vi "Facade Graph.vi"(0 "Data In":T4, 2 "Display State In":T2, 3 "Container State":T3) -> (6 "Data Out":T4, 7 "Display State Out":T2, 8 "Action":T1)   [LabVIEW 2009, in "Xgraph simple.xctl"]
doc: "Demonstration of an XControl.\n\nAAL 9/09"
uses:
  Xgraph simple.xctl
  Data Graph.ctl
  <vilib>/_xctls/Container State.ctl
  State Graph.ctl
  <vilib>/_xctls/Action.ctl
  <vilib>/_xctls/XControlSupport.lvlib
panel:
  in  "Plot Colors":u32[](array[colorbox])
  out "Xgraph simple":dbl[][](graph)
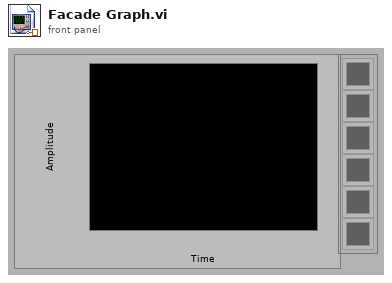
[diagram p1: front panel]
types:
  T1 = typedef "XControlSupport.lvlib/Action.ctl" = cluster{"Data Changed?":bool, "State Changed?":bool, "Action Name":string}
  T2 = typedef "Xgraph simple.xctl/State Graph.ctl" = cluster{"Show Points?":bool}
  T3 = typedef "XControlSupport.lvlib/Container State.ctl" = cluster{"Indicator?":bool, "Run Mode?":bool, " Refnum":refnum<vi>}
  T4 = typedef "Xgraph simple.xctl/Data Graph.ctl" = dbl[][]
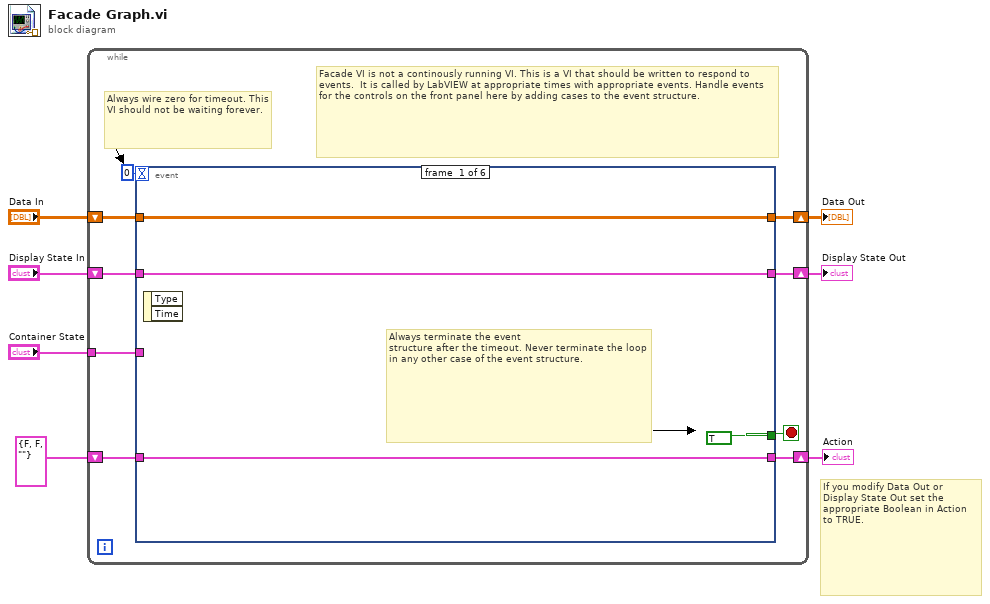
[diagram p0: block diagram]
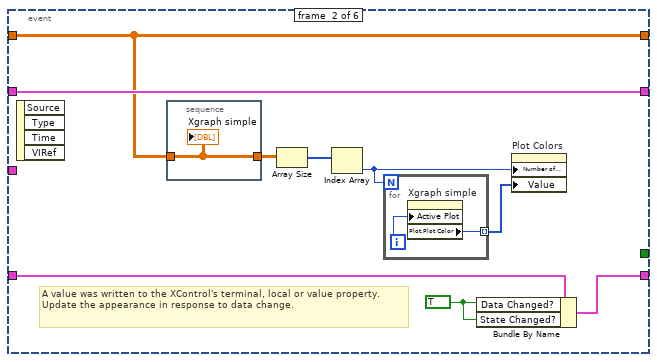
[diagram p2: hidden frame]
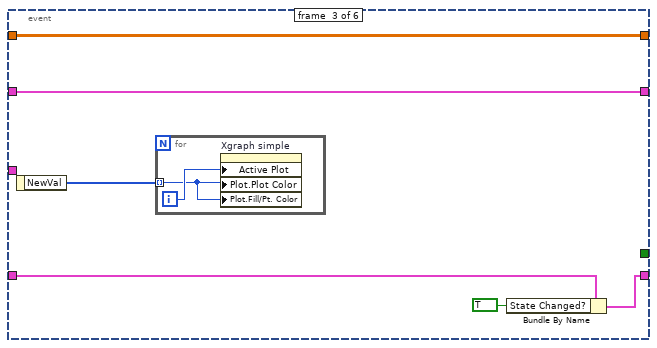
[diagram p3: hidden frame]
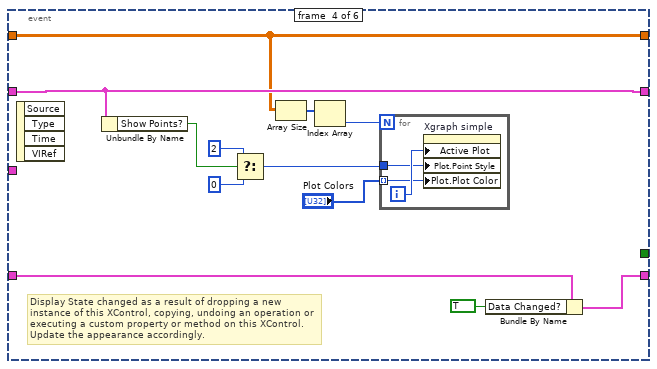
[diagram p4: hidden frame]
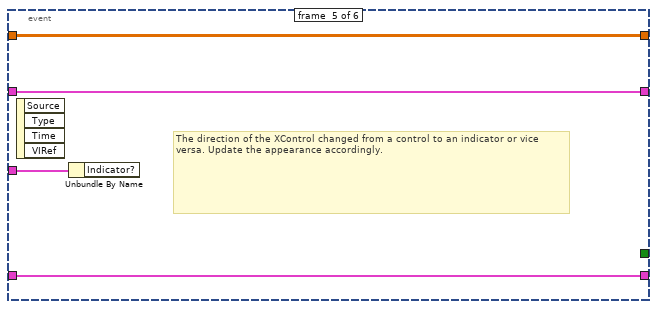
[diagram p5: hidden frame]
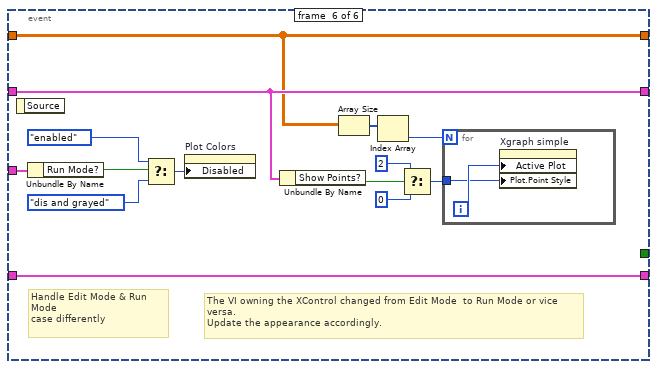
[diagram p6: hidden frame]
diagram:
  # "If you modify Data Out or\nDisplay State Out set the\nappropriate Boolean in Action\nto TRUE."
  n1 = while {
    shift-right: [w15] -> w4
    shift-left: "Display State In" -> [w16]
    tunnel: "Container State" -> [w12]
    shift-right: [w10] -> w7
    shift-left: "Data In" -> [w11]
    shift-right: [w8] -> w2
    shift-left: T1 {"Data Changed?"=FALSE, "State Changed?"=FALSE, "Action Name"=""} ("Action") -> [w9]
    stop <- w14 stop-if-true
    # "Facade VI is not a continously running VI. This is a VI that should be written to respond to events.  It is called by LabVIEW at appropriate times with appropriate events. Handle events for the controls on the front panel here by adding cases to the event structure."
    # "Always wire zero for timeout. This\nVI should not be waiting forever."
    n2 = event shown="[5] Exec State Change" {
      selector: _ -> [_ _ _ _ _ _]
      dyn-events: _ -> [_ _ _ _ _ _]
      timeout: 0 -> [_ _ _ _ _ _]
      tunnel: w16 -> [w18 w29 w33 w49 w58 w61]
      tunnel: [w18 w29 w33 w49 w58 w61] -> w15
      tunnel: [TRUE _ _ _ _ _] -> w14
      tunnel: w12 -> [_ _ _ _ w59 w73]
      tunnel: w11 -> [w17 w24 w35 w48 w57 w60]
      tunnel: [w17 w24 w35 w48 w57 w60] -> w10
      tunnel: [w19 w27 w37 w51 w56 w72] -> w8
      tunnel: w9 -> [w19 w28 w38 w52 w56 w72]
      event #0 {
        # "Always terminate the event\nstructure after the timeout. Never terminate the loop in any other case of the event structure."
        n3 = event-data() -> ()  [unwired: 1 in, 2 out]
      }
      event #1 {
        w26 = TRUE ("Data Changed?")
        # "A value was written to the XControl's terminal, local or value property.\nUpdate the appearance in response to data change."
        n4 = event-data() -> ()  [unwired: 1 in, 4 out]
        n5 = stacked-sequence {
          tunnel: w24 -> [w32]
          tunnel: [w32] -> w23
          frame #0 {
            "Xgraph simple" <- w32
          }
        }
        n6 = Array Size(array=w23) -> (size(s)=w25:i32[])
        n7 = Index Array(array=w25) -> (element=w22:i32)  [unwired: 1 in]
        n8 = for {
          N: w22 -> [_]
          tunnel: [w30] -> w21 mode=indexing
          i -> [w31]
          n9 = property on="Xgraph simple" class="WFGraph (strict)"("Active Plot"=w31) -> ("Plot.Plot Color"=w30:u32)  [unwired: 2 in, 2 out]
        }
        n10 = Bundle By Name(cluster=w28, "Data Changed?"=w26, "State Changed?"=w26) -> (w27:T1)
        n11 = property on="Plot Colors" class="Arr (strict)"("Number of Rows"=w22, "Value"=w21) -> ()  [unwired: 2 in, 2 out]
      }
      event #2 {
        n12 = event-data() -> ("NewVal"=w34:u32[])  [unwired: 1 in]
        n13 = for {
          tunnel: w34 -> [w39] mode=indexing
          i -> [w40]
          n14 = property on="Xgraph simple" class="WFGraph (strict)"("Active Plot"=w40, "Plot.Plot Color"=w39, "Plot.Fill/Pt. Color"=w39) -> ()  [unwired: 2 in, 2 out]
        }
        n15 = Bundle By Name(cluster=w38, "State Changed?"=TRUE) -> (w37:T1)
      }
      event #3 {
        # "Display State changed as a result of dropping a new instance of this XControl, copying, undoing an operation or executing a custom property or method on this XControl. Update the appearance accordingly."
        n16 = event-data() -> ()  [unwired: 1 in, 4 out]
        n17 = Unbundle By Name(w49) -> ("Show Points?"=w45:bool)
        n18 = Select(t=2, s=w45, f=0) -> (s? t:f=w42:i32)
        n19 = Array Size(array=w48) -> (size(s)=w47:i32[])
        n20 = Index Array(array=w47) -> (element=w46:i32)  [unwired: 1 in]
        n21 = for {
          N: w46 -> [_]
          tunnel: w42 -> [w54]
          tunnel: "Plot Colors" -> [w53] mode=indexing
          i -> [w55]
          n22 = property on="Xgraph simple" class="WFGraph (strict)"("Active Plot"=w55, "Plot.Point Style"=w54, "Plot.Plot Color"=w53) -> ()  [unwired: 2 in, 2 out]
        }
        n23 = Bundle By Name(cluster=w52, "Data Changed?"=TRUE) -> (w51:T1)
      }
      event #4 {
        # "The direction of the XControl changed from a control to an indicator or vice versa. Update the appearance accordingly."
        n24 = event-data() -> ()  [unwired: 1 in, 4 out]
        n25 = Unbundle By Name(w59) -> ()  [unwired: 1 out]
      }
      event #5 {
        # "The VI owning the XControl changed from Edit Mode  to Run Mode or vice versa.\nUpdate the appearance accordingly."
        # "Handle Edit Mode & Run Mode\ncase differently"
        n26 = event-data() -> ()  [unwired: 1 in, 1 out]
        n27 = Unbundle By Name(w73) -> ("Run Mode?"=w71:bool)
        n28 = Select(t=enum16{"enabled", "disabled", "dis and grayed"}."enabled", s=w71, f=enum16{"enabled", "disabled", "dis and grayed"}."dis and grayed") -> (s? t:f=w69:enum16{"enabled", "disabled", "dis and grayed"})
        n29 = property on="Plot Colors" class="Arr (strict)"("Disabled"=w69) -> ()  [unwired: 2 in, 2 out]
        n30 = Unbundle By Name(w61) -> ("Show Points?"=w65:bool)
        n31 = Array Size(array=w60) -> (size(s)=w67:i32[])
        n32 = Index Array(array=w67) -> (element=w66:i32)  [unwired: 1 in]
        n33 = Select(t=2, s=w65, f=0) -> (s? t:f=w62:i32)
        n34 = for {
          N: w66 -> [_]
          tunnel: w62 -> [w74]
          i -> [w75]
          n35 = property on="Xgraph simple" class="WFGraph (strict)"("Active Plot"=w75, "Plot.Point Style"=w74) -> ()  [unwired: 2 in, 2 out]
        }
      }
    }
  }
  "Display State Out" <- w4
  "Data Out" <- w7
  "Action" <- w2
